vi "数据优化.vi"(3 "图像簇":T2, 4 "光源散斑簇":T3, 5 "模块选择簇":T1) -> (0 "散斑图像作用结果优化":dbl[](array[numeric]), 1 "优化光源散斑簇":T3, 2 "优化图像簇":T2)   [LabVIEW 2018]
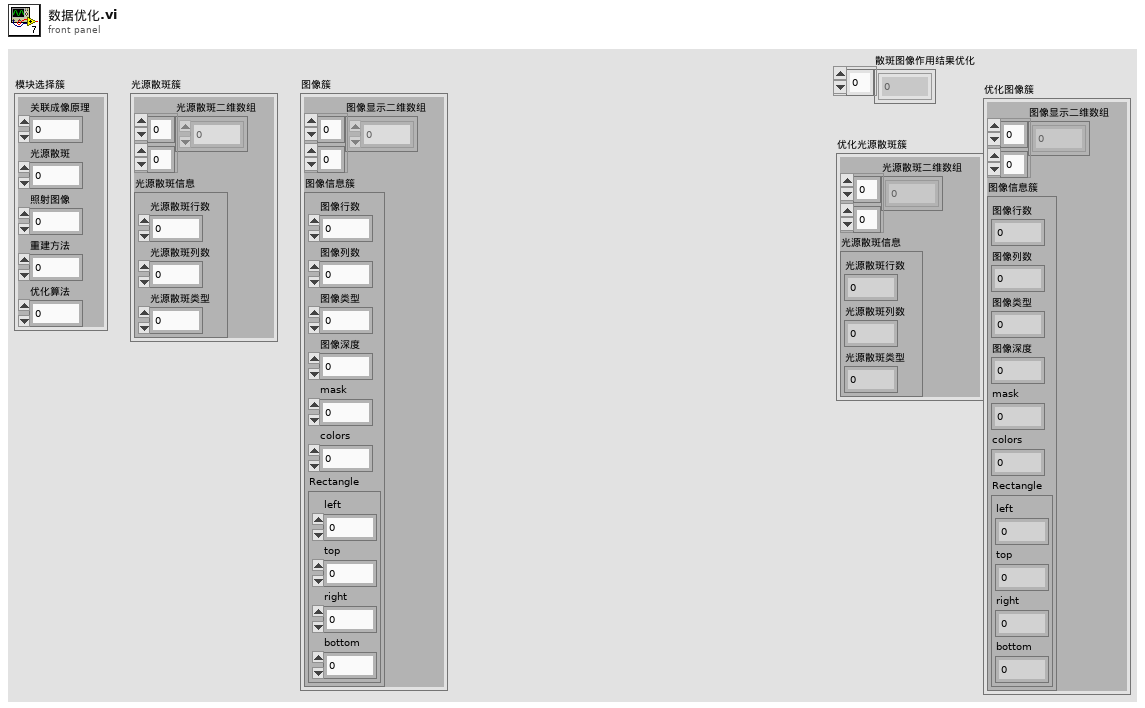
[diagram p1: front panel]
types:
  T1 = cluster{"关联成像原理":i32, "光源散斑":i32, "照射图像":i32, "重建方法":i32, "优化算法":i32}
  T2 = cluster{"图像显示二维数组":dbl[][], "图像信息簇":cluster{"图像行数":dbl, "图像列数":dbl, "图像类型":dbl, "图像深度":i32, "mask":i32, "colors":i32, "Rectangle":cluster{"left":i16, "top":i16, "right":i16, "bottom":i16}}}
  T3 = cluster{"光源散斑二维数组":dbl[][], "光源散斑信息":cluster{"光源散斑行数":dbl, "光源散斑列数":dbl, "光源散斑类型":dbl}}
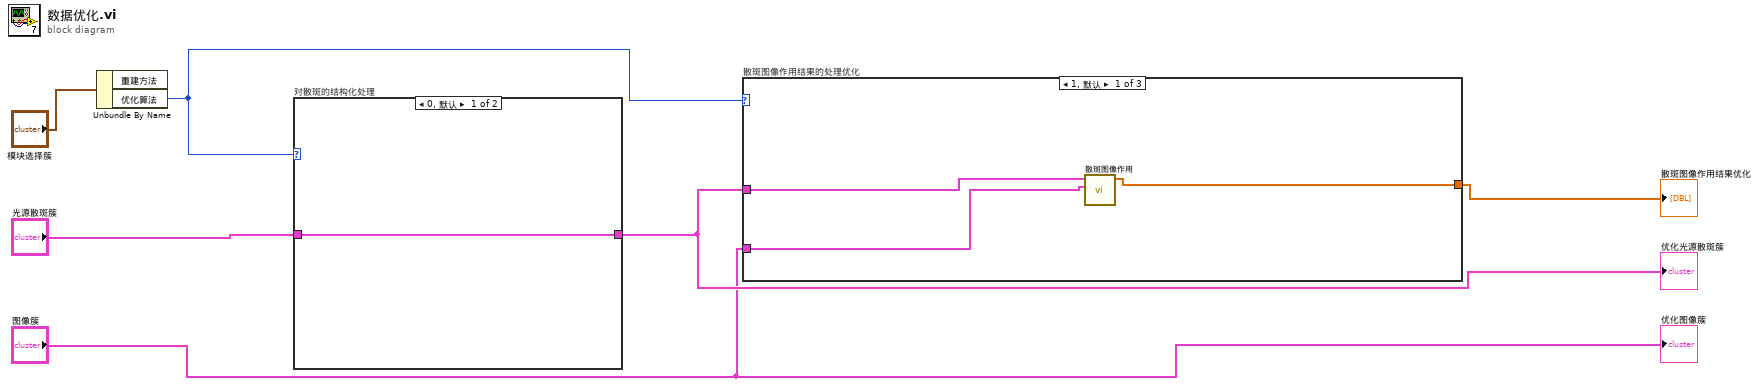
[diagram p0: block diagram]
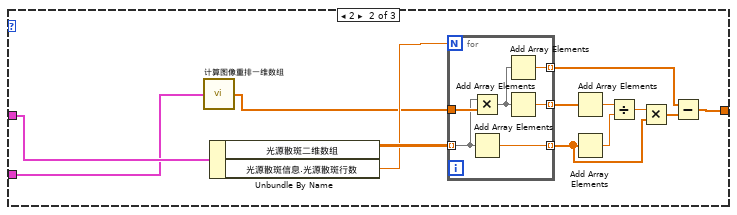
[diagram p3: hidden frame]
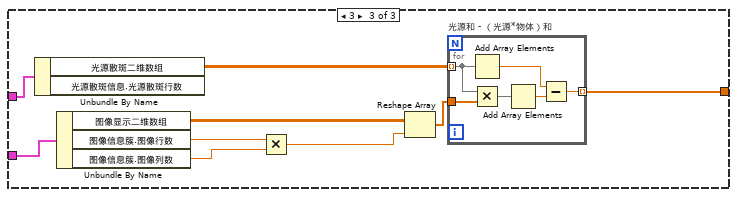
[diagram p4: hidden frame]
diagram:
  n1 = Unbundle By Name("模块选择簇") -> ("优化算法"=w2:i32)  [unwired: 1 out]
  n2 = case "对散斑的结构化处理" shown="0, 默认" w2 {
    tunnel: [w7 w8] -> w5
    tunnel: "光源散斑簇" -> [w7 w8]
    frame 0, Default {
    }
    frame 1 {
    }
  }
  "优化光源散斑簇" <- w5
  n3 = case "散斑图像作用结果的处理优化" shown="1, 默认" w2 {
    tunnel: "图像簇" -> [w10 w13 w35]
    tunnel: w5 -> [w11 w15 w34]
    tunnel: [w9 w16 w31] -> w1
    frame 1, Default {
      n4 = call "散斑图像作用.vi"("图像簇"=w10, "光源散斑簇"=w11) -> ("散斑图像作用聚焦数组"=w9:dbl[])  [unwired: 9 in]
    }
    frame 2 {
      n5 = call "计算图像重排一维数组.vi"("优化图像簇"=w13) -> ("图像重排一维数组"=w12:dbl[])
      n6 = Unbundle By Name(w15) -> ("光源散斑二维数组"=w21:dbl[][], "光源散斑信息.光源散斑行数"=w17:dbl)
      n7 = for {
        N: w17 -> [_]
        tunnel: w21 -> [w28] mode=indexing
        tunnel: w12 -> [w30]
        tunnel: [w29] -> w18 mode=indexing
        tunnel: [w27] -> w14 mode=indexing
        tunnel: [w25] -> w23 mode=indexing
        n8 = Multiply(x=w28, y=w30) -> (x*y=w26:dbl[])
        n9 = Add Array Elements(numeric array=w28) -> (sum=w27:dbl)
        n10 = Add Array Elements(numeric array=w26) -> (sum=w25:dbl)
        n11 = Add Array Elements(numeric array=w26) -> (sum=w29:dbl)
      }
      n12 = Add Array Elements(numeric array=w18) -> (sum=w19:dbl)
      n13 = Add Array Elements(numeric array=w14) -> (sum=w20:dbl)
      n14 = Divide(x=w19, y=w20) -> (x/y=w22:dbl)
      n15 = Multiply(x=w22, y=w14) -> (x*y=w24:dbl[])
      n16 = Subtract(x=w23, y=w24) -> (x-y=w16:dbl[])
    }
    frame 3 {
      n17 = Unbundle By Name(w34) -> ("光源散斑二维数组"=w33:dbl[][])  [unwired: 1 out]
      n18 = Unbundle By Name(w35) -> ("图像显示二维数组"=w36:dbl[][], "图像信息簇.图像行数"=w37:dbl, "图像信息簇.图像列数"=w38:dbl)
      n19 = Multiply(x=w37, y=w38) -> (x*y=w39:dbl)
      n20 = Reshape Array(w36, w39) -> (w32:dbl[])
      n21 = for "光源和 - （光源*物体）和" {
        tunnel: w33 -> [w40] mode=indexing
        tunnel: w32 -> [w45]
        tunnel: [w42] -> w31 mode=indexing
        n22 = Add Array Elements(numeric array=w40) -> (sum=w41:dbl)
        n23 = Multiply(x=w40, y=w45) -> (x*y=w44:dbl[])
        n24 = Add Array Elements(numeric array=w44) -> (sum=w43:dbl)
        n25 = Subtract(x=w41, y=w43) -> (x-y=w42:dbl)
      }
    }
  }
  "散斑图像作用结果优化" <- w1
  "优化图像簇" <- "图像簇"
